vi "Polling Interval.vi"(8 "error in (no error)":errorcluster, 10 "Polling Interval":dbl[unit], 11 "CS++BaseActor in":refnum<class "CS++BaseActor.lvclass">) -> (0 "error out":errorcluster, 3 "CS++BaseActor out":refnum<class "CS++BaseActor.lvclass">)   [LabVIEW 2015, in "CS++BaseActor.lvlib" / "CS++BaseActor.lvclass"]
doc: "Intervall for periodic actions.\n\n<b>Attention:</b> Be aware of message pileup if intervall is too short."
uses:
  CS++BaseActor.lvclass
  CS++BaseActor.lvclass/CS++BaseActor.ctl
  <vilib>/ActorFramework/Actor/Actor.lvclass/Actor.ctl
  <vilib>/ActorFramework/Message Enqueuer/Message Enqueuer.lvclass/Message Enqueuer.ctl
  CS++BaseActor Messages/Polling Start Stop Msg/Polling Start Stop Msg.lvclass/Polling Start Stop Msg.ctl
  <vilib>/ActorFramework/Message Enqueuer/Init from Existing Queue.vi
  <vilib>/ActorFramework/Message Enqueuer/Enqueue.vi
  <vilib>/ActorFramework/Message Priority Queue/Priority Enqueue.vi
  CS++BaseActor Messages/Polling Start Stop Msg/Polling Start Stop Msg.lvclass
  <vilib>/ActorFramework/Message Enqueuer/Message Enqueuer.lvclass
  <vilib>/ActorFramework/Actor/Actor.lvclass
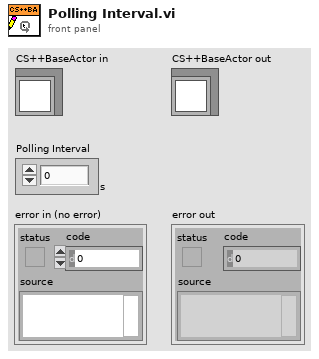
[diagram p1: front panel]
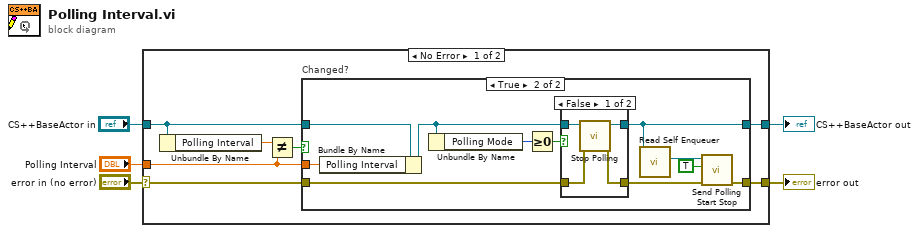
[diagram p0: block diagram]
diagram:
  n1 = case shown="No Error" "error in (no error)" {
    selector: "error in (no error)" -> [w7 w32]
    tunnel: [w6 w32] -> w4
    tunnel: [w12 w33] -> w2
    tunnel: "CS++BaseActor in" -> [w11 w33]
    tunnel: "Polling Interval" -> [w9 _]
    frame No Error {
      n2 = Unbundle By Name(w11) -> ("Polling Interval"=w10:dbl[unit])
      n3 = Not Equal?(x=w10, y=w9) -> (x != y?=w8:bool)
      n4 = case "Changed?" shown="True" w8 {
        tunnel: [w14 w19] -> w12
        tunnel: w11 -> [w14 w21]
        tunnel: w9 -> [_ w22]
        tunnel: w7 -> [w13 w23]
        tunnel: [w13 w17] -> w6
        frame False {
        }
        frame True {
          n5 = Bundle By Name(cluster=w21, "Polling Interval"=w22) -> (w20:refnum<class "CS++BaseActor.lvclass">)
          n6 = Unbundle By Name(w20) -> ("Polling Mode"=w25:i32)
          n7 = Greater Or Equal To 0?(x=w25) -> (x >= 0?=w24:bool)
          n8 = case shown="False" w24 {
            tunnel: [w28 w31] -> w19
            tunnel: w20 -> [w29 w31]
            tunnel: w23 -> [w27 w30]
            tunnel: [w26 w30] -> w18
            frame False {
              n9 = call "Stop Polling.vi"("Error In"=w27, "CS++BaseActor in"=w29) -> ("Error Out"=w26:errorcluster, "CS++BaseActor out"=w28:refnum<class "CS++BaseActor.lvclass">)  [unwired: 8 in]
            }
            frame True {
            }
          }
          n10 = call <vilib>:"Read Self Enqueuer.vi"("Actor"=w19) -> ("Self Enqueuer"=w16:refnum<class "Message Enqueuer.lvclass">)  [unwired: 10 in]
          n11 = call "Send Polling Start Stop.vi"("error in (no error)"=w18, "Start Polling"=TRUE, "Message Enqueuer"=w16) -> ("error out"=w17:errorcluster)  [unwired: 7 in, 1 out]
        }
      }
    }
    frame Error {
    }
  }
  "error out" <- w4
  "CS++BaseActor out" <- w2
